vi "Limit value.vi"(1 "Current Value in":i32, 8 "max undo steps":i32) -> (15 "Value out":i32)   [LabVIEW 2012]
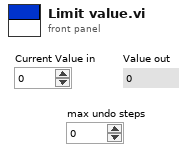
[diagram p1: front panel]
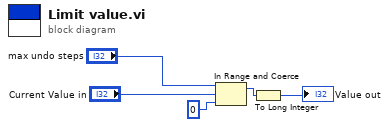
[diagram p0: block diagram]
diagram:
  n1 = In Range and Coerce(upper limit="max undo steps", x="Current Value in", lower limit=0) -> (coerced(x)=w3:i32)  [unwired: 1 out]
  n2 = To Long Integer(number=w3) -> (32bit integer=→"Value out":i32)
